vi "Module Loop.vi"(8 "error in (no error)":errorcluster, 11 "Remote Messaging Module in":refnum<class "Remote Messaging Module.lvclass">) -> (0 "error out":errorcluster, 3 "Remote Messaging Module out":refnum<class "Remote Messaging Module.lvclass">)   [LabVIEW 2020, in "Volatus.lvlib" / "Remote Messaging Module.lvclass"]
uses:
  Remote Messaging Module.lvclass
  Remote Messaging Module.lvclass/Remote Messaging Module.ctl
  Module/Module.lvclass
  C:/dev/lv20CE/relink/lv-volatus/Volatus/Module/Module.lvclass
  C:/dev/lv20CE/relink/lv-volatus/Volatus/Remote Messaging Module/Remote Messaging Module.lvclass
  lv-vecto/Vecto/proto/TcpPayload/Data.ctl
  lv-vecto/Vecto/proto/TcpPayload/TcpPayload.lvlib
  MessageQ/MessageQ.lvclass
  Message Registration.ctl
  Messages Registration.ctl
  Message Unregistration.ctl
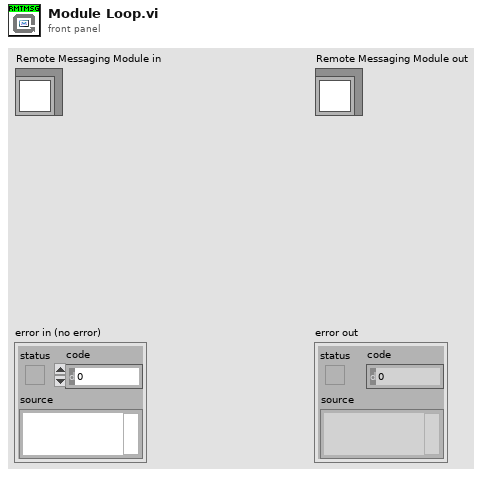
[diagram p1: front panel]
types:
  T1 = typedef "TcpPayload.lvlib/Data.ctl" = cluster{"target_node":u32, "source_id":u32, "sequence":u32, "timestamp":u64, "type":string, "task_id":string, "payload":u8[]}
  T2 = typedef "Volatus.lvlib/Remote Messaging Module.lvclass/Messages Registration.ctl" = cluster{"MessageQ":refnum<class "MessageQ.lvclass">, "Messages":T3[]}
  T3 = typedef "Volatus.lvlib/Remote Messaging Module.lvclass/Message Registration.ctl" = cluster{"Message Type":string, "Message ID":string}
  T4 = typedef "Volatus.lvlib/Remote Messaging Module.lvclass/Message Unregistration.ctl" = cluster{"MessageQ":refnum<class "MessageQ.lvclass">}
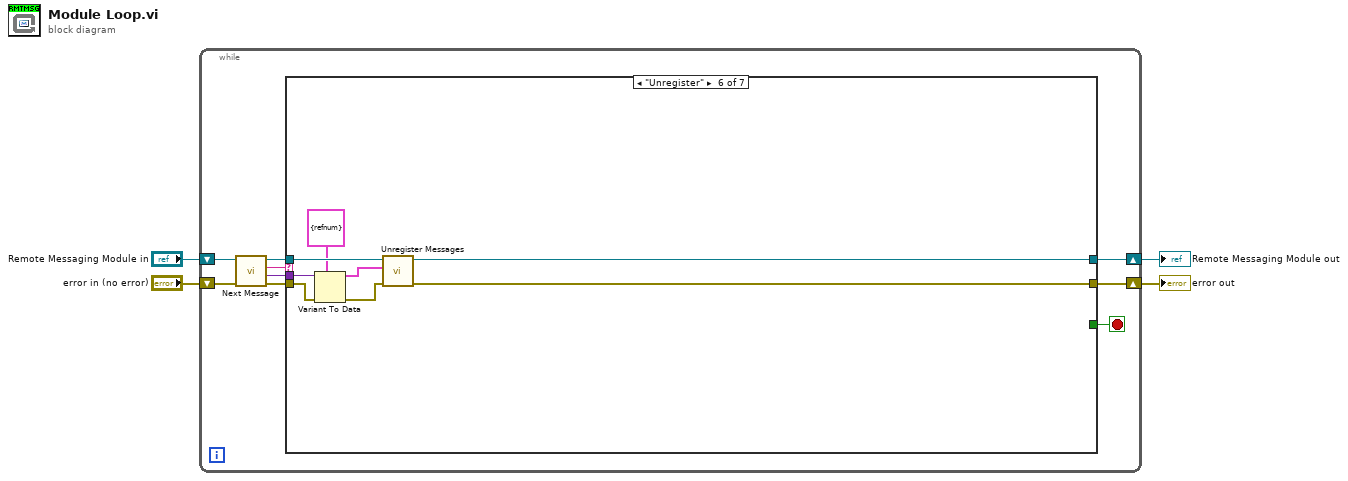
[diagram p0: block diagram]
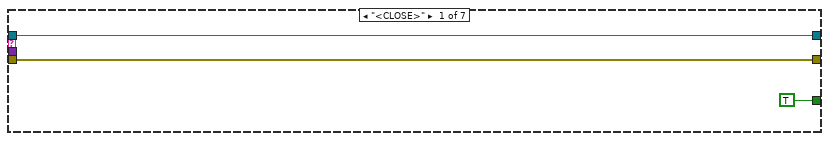
[diagram p2: hidden frame]
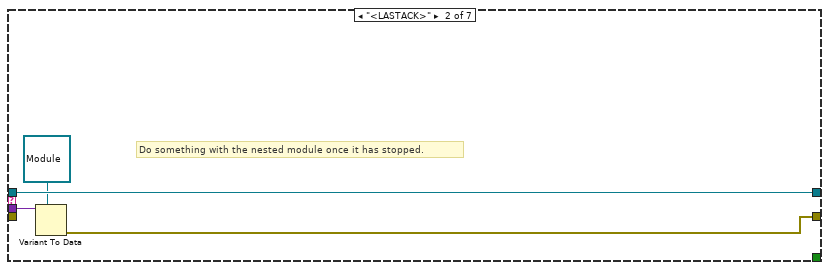
[diagram p3: hidden frame]
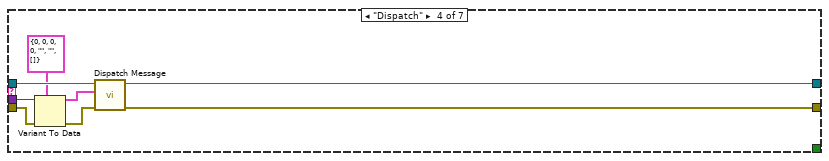
[diagram p5: hidden frame]
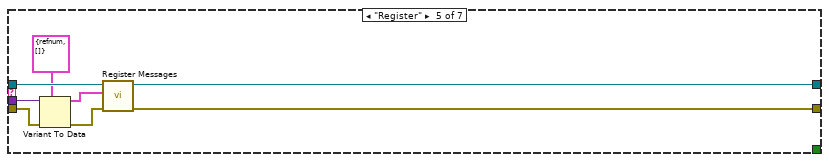
[diagram p6: hidden frame]
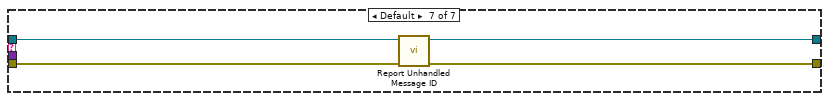
[diagram p7: hidden frame]
diagram:
  n1 = while {
    shift-right: [w8] -> w1
    shift-left: "Remote Messaging Module in" -> [w13]
    shift-right: [w7] -> w2
    shift-left: "error in (no error)" -> [w12]
    stop <- w6 stop-if-true
    n2 = call "Next Message.vi"("error in (no error)"=w12, "Module in"=w13) -> ("error out"=w11:errorcluster, "Data"=w5:variant, "ID"=w10:string, "Module out"=w9:refnum<class "Remote Messaging Module.lvclass">)  [unwired: 6 in]
    n3 = case shown="\"Unregister\"" w10 {
      tunnel: w11 -> [w14 _ w21 w28 w36 w45 w50]
      tunnel: w9 -> [w15 w20 w22 w30 w38 w46 w48]
      tunnel: [w15 w20 w22 w26 w34 w42 w47] -> w8
      tunnel: [w14 w17 w21 w23 w31 w40 w49] -> w7
      tunnel: [TRUE _ _ _ _ _ _] -> w6
      tunnel: w5 -> [_ w19 _ w29 w37 w44 _]
      frame "<CLOSE>" {
      }
      frame "<LASTACK>" {
        # "Do something with the nested module once it has stopped."
        n4 = Variant To Data(type=refnum<class "Module.lvclass"> refnum ("Volatus:Module"), Variant=w19) -> (error out=w17:errorcluster)  [unwired: 1 in, 1 out]
      }
      frame "<TIMEOUT>" {
        # "No message for this module was received in time"
      }
      frame "Dispatch" {
        n5 = Variant To Data(error in=w28, type=T1 {"target_node"=0, "source_id"=0, "sequence"=0, "timestamp"=0, "type"="", "task_id"="", "payload"=[]} ("TcpPayload"), Variant=w29) -> (data=w25:T1, error out=w24:errorcluster)
        n6 = call "Dispatch Message.vi"("error in (no error)"=w24, "TcpPayload"=w25, "Remote Messaging Module in"=w30) -> ("error out"=w23:errorcluster, "Remote Messaging Module out"=w26:refnum<class "Remote Messaging Module.lvclass">)  [unwired: 7 in]
      }
      frame "Register" {
        n7 = Variant To Data(error in=w36, type=T2 {"MessageQ"=refnum, "Messages"=[]} ("Messages Registration"), Variant=w37) -> (data=w33:T2, error out=w32:errorcluster)
        n8 = call "Register Messages.vi"("error in (no error)"=w32, "Messages Registration"=w33, "Remote Messaging Module in"=w38) -> ("error out"=w31:errorcluster, "Remote Messaging Module out"=w34:refnum<class "Remote Messaging Module.lvclass">)  [unwired: 7 in]
      }
      frame "Unregister" {
        n9 = Variant To Data(error in=w45, type=T4 {"MessageQ"=refnum} ("Message Unregistration"), Variant=w44) -> (data=w39:T4, error out=w41:errorcluster)
        n10 = call "Unregister Messages.vi"("error in (no error)"=w41, "Message Unregistration"=w39, "Remote Messaging Module in"=w46) -> ("error out"=w40:errorcluster, "Remote Messaging Module out"=w42:refnum<class "Remote Messaging Module.lvclass">)  [unwired: 7 in]
      }
      frame Default {
        n11 = call "Report Unhandled Message ID.vi"("error in (no error)"=w50, "Module in"=w48) -> ("error out"=w49:errorcluster, "Module out"=w47:refnum<class "Remote Messaging Module.lvclass">)  [unwired: 8 in]
      }
    }
  }
  "error out" <- w2
  "Remote Messaging Module out" <- w1
